vi "Drive Threshold and Half.vi"(5 "Send to DB Name":string="Numeric Array", 7 "Drive refnum name":string="RobotDrive", 8 "Speed Toggle":bool, 9 "R In":dbl, 10 "Y In":dbl, 11 "X In":dbl) -> ()   [LabVIEW 2014]
uses:
  <vilib>/Rock Robotics/WPI/RobotDrive/WPI_RobotDriveGetSetRefNum.vi
  <vilib>/Rock Robotics/WPI/RobotDrive/WPI_RobotDriveMecanumDrive_Cartesian.vi
  <vilib>/Rock Robotics/Network Tables/SD Write Numeric Array.vi
panel:
  out "X Original":dbl
  out "X Threshold":dbl
  out "Y Original":dbl
  out "Y Threshold":dbl
  out "R Original":dbl
  out "R Threshold":dbl
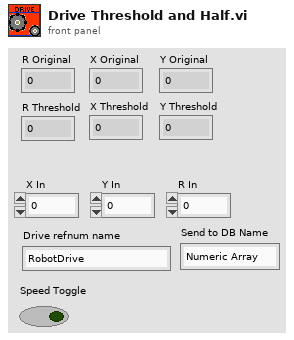
[diagram p1: front panel]
types:
  T1 = typedef "WPI_RobotDriveDevRef.ctl" = cluster{"DevStatus":errorcluster, "Motors[]":T2[], "Square Inputs":bool, "Max Output":dbl}
  T2 = typedef "WPI_MotorControlDeviceRef.ctl" = cluster{"DeviceStatus":errorcluster, "Type":T3, "PWM":cluster{"Controller":T4, "PWM Channel":T5, "DeadBand":T6}, "CAN":cluster{"Device Number":u8, "Control Mode":T7, "Semaphore":T8, "Max Vout":dbl, "TalonSRX Control Mode":T9}, "Invert":bool, "TransformRef":T10, "InvTransformRef":T10}
  T3 = typedef "WPI_MotorControlType.ctl" = enum16{"PWM", "CAN", "CANTalonSRX"}
  T4 = typedef "FPGA_TypedefDigitalModule.ctl" = enum16{"Controller 1"}
  T5 = typedef "FPGA_DIOPWMChannel.ctl" = enum8{"PWM 0", "PWM 1", "PWM 2", "PWM 3", "PWM 4", "PWM 5", "PWM 6", "PWM 7", "PWM 8", "PWM 9", "PWM MXP 0", "PWM MXP 1", "PWM MXP 2", "PWM MXP 3", "PWM MXP 4", "PWM MXP 5", "PWM MXP 6", "PWM MXP 7", "PWM MXP 8", "PWM MXP 9", "Invalid"}
  T6 = typedef "WPI_PWMDeadband.ctl" = cluster{"Name":string, "maxPositivePwm":i32, "minPositivePwm":i32, "centerPwm":i32, "maxNegativePwm":i32, "minNegativePwm":i32, "angularRange":u16}
  T7 = typedef "WPI_CANJaguar_ControlMode.ctl" = enum8{"Percent VBus", "Current", "Speed", "Position", "Voltage"}
  T8 = typedef "Semaphore RefNum" = refnum<k1>
  T9 = typedef "WPI_CANTalonSRX_APIControlMode.ctl" = enum8{"Percent VBus", "Speed", "Position", "Slave", "Unchanged / Invalid"}
  T10 = typedef "WPI_PWMTransform_ConPane.ctl" = refnum<vi>
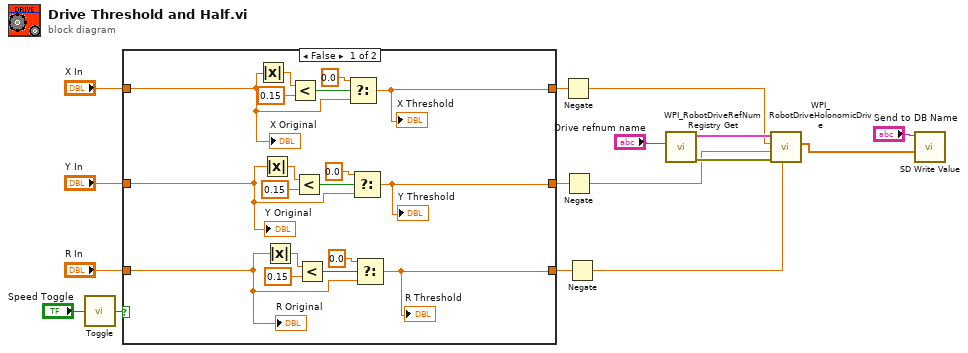
[diagram p0: block diagram]
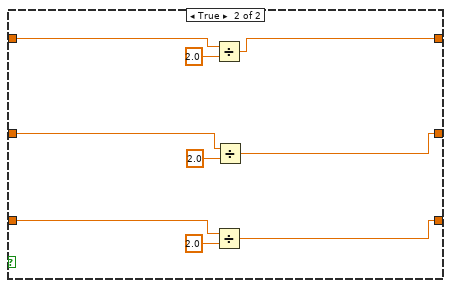
[diagram p2: hidden frame]
diagram:
  n1 = call "Toggle.vi"("Input"="Speed Toggle") -> ("Output"=w16:bool)
  n2 = case shown="False" w16 {
    tunnel: [w29 w37] -> w15
    tunnel: "X In" -> [w30 w38]
    tunnel: "Y In" -> [w24 w39]
    tunnel: [w23 w36] -> w10
    tunnel: "R In" -> [w18 w40]
    tunnel: [w17 w35] -> w9
    frame False {
      n3 = Absolute Value(x=w30) -> (abs(x)=w34:dbl)
      n4 = Absolute Value(x=w24) -> (abs(x)=w28:dbl)
      n5 = Absolute Value(x=w18) -> (abs(x)=w19:dbl)
      n6 = Less?(x=w34, y=0.15) -> (x < y?=w32:bool)
      n7 = Less?(x=w28, y=0.15) -> (x < y?=w26:bool)
      n8 = Less?(x=w19, y=0.15) -> (x < y?=w21:bool)
      n9 = Select(t=0.0, s=w32, f=w30) -> (s? t:f=w29:dbl)
      "X Threshold" <- w29
      n10 = Select(t=0.0, s=w26, f=w24) -> (s? t:f=w23:dbl)
      "Y Threshold" <- w23
      n11 = Select(t=0.0, s=w21, f=w18) -> (s? t:f=w17:dbl)
      "R Threshold" <- w17
      "X Original" <- w30
      "Y Original" <- w24
      "R Original" <- w18
    }
    frame True {
      n12 = Divide(x=w38, y=2.0) -> (x/y=w37:dbl)
      n13 = Divide(x=w40, y=2.0) -> (x/y=w35:dbl)
      n14 = Divide(x=w39, y=2.0) -> (x/y=w36:dbl)
    }
  }
  n15 = Negate(x=w15) -> (-x=w3:dbl)
  n16 = Negate(x=w10) -> (-x=w2:dbl)
  n17 = Negate(x=w9) -> (-x=w1:dbl)
  n18 = call <vilib>:"WPI_RobotDriveRefNum Registry Get.vi"("refnum name"="Drive refnum name") -> ("error out"=w8:errorcluster, "RobotDriveDevRef"=w7:T1)  [unwired: 9 in]
  n19 = call-poly <vilib>:"WPI_RobotDriveHolonomicDrive.vi"("Rotation"=w1, "error in (no error)"=w8, "Y"=w2, "X"=w3, "RobotDriveDevRef"=w7) -> ("Motor Values"=w6:dbl[])  [unwired: 4 in, 2 out]
  n20 = call-poly <vilib>:"SD Write Value.vi"("Numeric Array"=w6, "Name"="Send to DB Name") -> ()  [unwired: 8 in, 2 out]
